vi "run inspection.vi"(7 "Results where TCF match":path[](array[path]), 8 "error in":errorcluster, 9 "Scans[]":T1(array[cluster]), 10 "APG Config":T8, 11 "Programming Data":T2) -> (0 "error out":errorcluster, 2 "Scans[]":T1(array[cluster]), 3 "Inspection passed":bool)   [LabVIEW 2013, in "Manipulate IPF.lvlib"]
uses:
  Manipulate IPF.lvlib
  Settings/type_def/APG Config.ctl
  type_def/files.ctl
  3013/code/Modules/Inspection/Data/Panel_class/type_def/Config File data.ctl
  3013/code/Modules/Inspection/type_def/Pos and Rot.ctl
  3013/code/Modules/Inspection/Data/PCB_class/type_def/PCB Params.ctl
  3013/code/Modules/Inspection/Data/Panel_class/type_def/BarCode Params.ctl
  3013/code/Modules/Barcode Reader/type_def/id.ctl
  <vilib>/addons/WireFlow/_WF_ProgressBar.llb/WindowBehavior.ctl
  <vilib>/addons/WireFlow/_WF_ProgressBar.llb/MessageTextType.ctl
  <vilib>/Utility/sysdir.llb/System Directory Type.ctl
  <vilib>/addons/WireFlow/_WF_ProgressBar.llb/ProgressBar_WireFlow.lvclass
  <userlib>/_OpenG.lib/file/file.llb/Convert File Extension (Path)__ogtk.vi
  <userlib>/_OpenG.lib/file/file.llb/File Exists - Scalar__ogtk.vi
  Mike/APG_mike a3Di.lvlib
  Debug Results/Debug Results.lvlib
  Settings/APG_settings.lvlib
  3013/code/Modules/Inspection/Inspection.lvlib
  3013/code/Modules/Inspection/Data/PCB_class/PCB.lvclass
  3013/code/Modules/Barcode Reader/Barcode Reader.lvlib
  3013/code/Modules/Inspection/Data/Panel_class/Panel.lvclass
  a3Di APG.lvlib
panel:
  out "Array 2":path[](array[path])
  out "Array":path[](array[path])
  out "standard output":string
  out "cmd line":string
  out "Comand debug":string
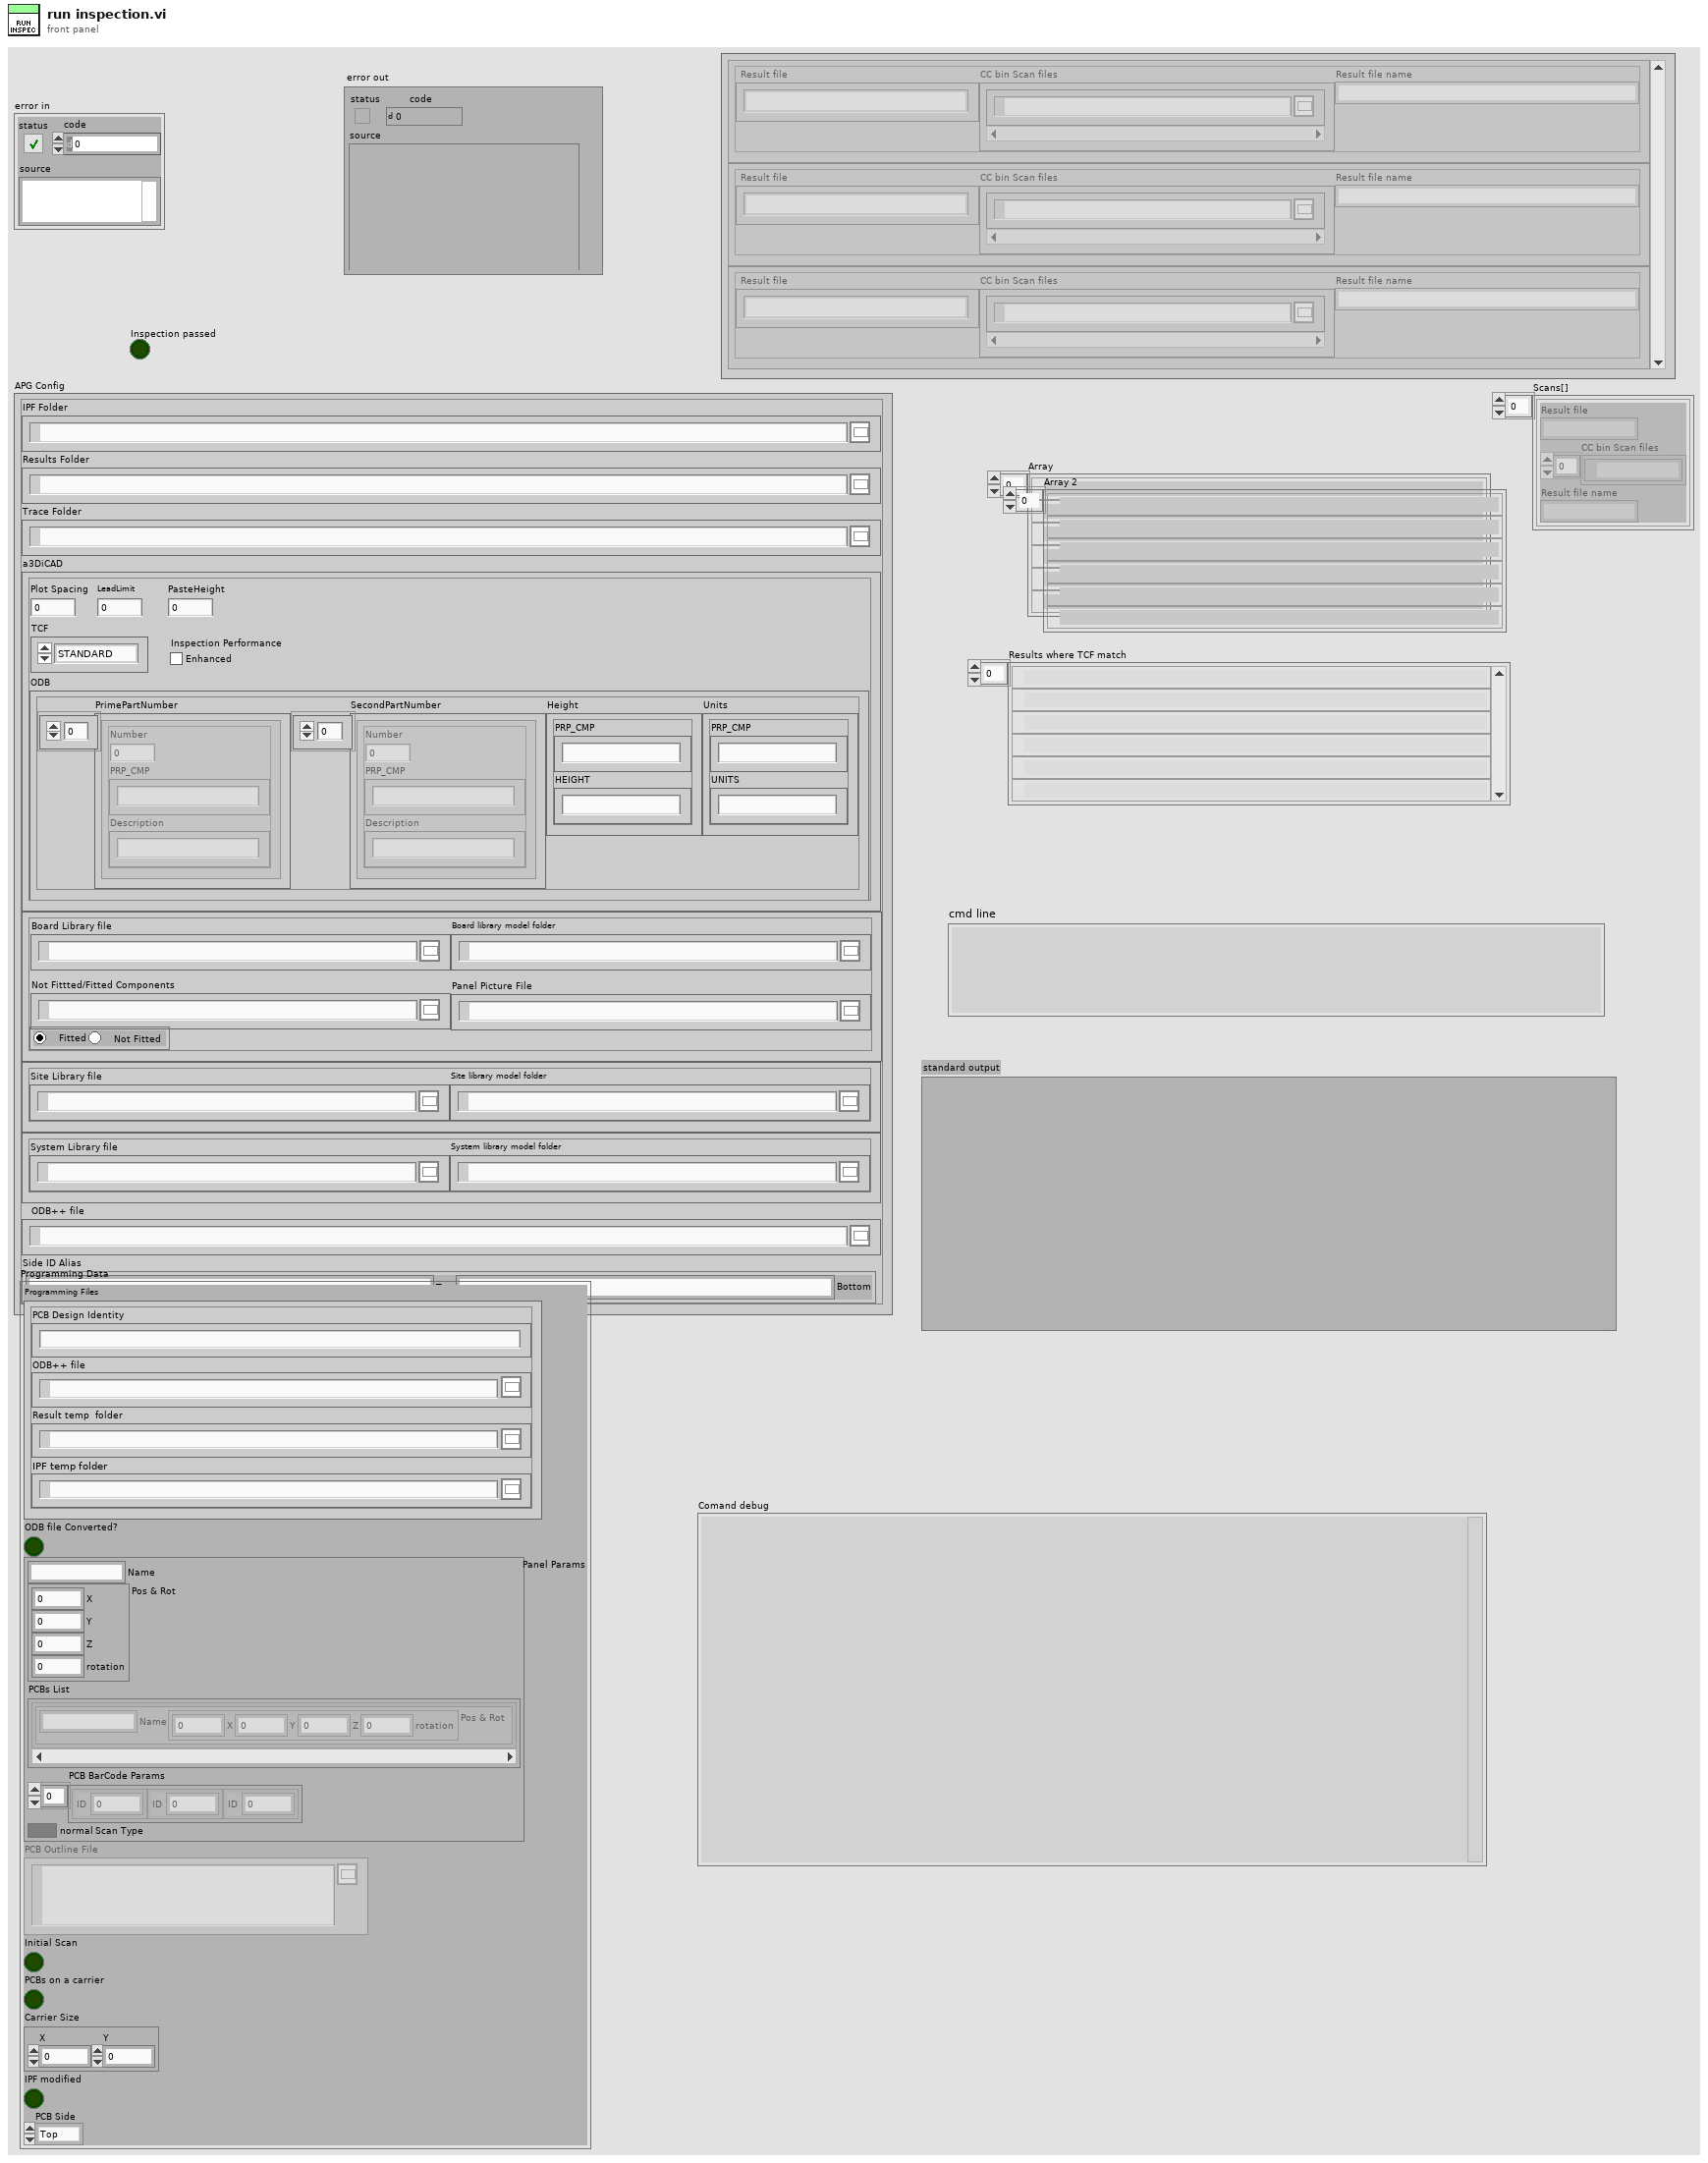
[diagram p1: front panel]
types:
  T1 = cluster{"Result file":string, "CC bin Scan files":path[], "Result file name":string}[]
  T2 = typedef "a3Di APG.lvlib/files.ctl" = cluster{"Programming Files":cluster{"PCB Design Identity":string, "ODB++ file":path, "Result temp  folder":path, "IPF temp folder":path}, "ODB file Converted?":bool, "Panel Params":T3, "PCB Outline File":path, "Initial Scan":bool, "PCBs on a carrier":bool, "Carrier Size":cluster{"X":dbl, "Y":dbl}, "IPF modified":bool, "PCB Side":enum16{"Top", "Bottom"}}
  T3 = typedef "Inspection.lvlib/Panel.lvclass/Config File data.ctl" = cluster{"Name":string, "Pos & Rot":T4, "PCBs List":cluster{"PCB Params":T5}[], "PCB BarCode Params":T6[], "Scan Type":bool}
  T4 = typedef "Inspection.lvlib/Pos and Rot.ctl" = cluster{"X":dbl, "Y":dbl, "Z":dbl, "rotation":dbl}
  T5 = typedef "Inspection.lvlib/PCB.lvclass/PCB Params.ctl" = cluster{"Name":string, "Pos & Rot":T4}
  T6 = typedef "Inspection.lvlib/Panel.lvclass/BarCode Params.ctl" = cluster{"ID":T7}
  T7 = typedef "Barcode Reader.lvlib/id.ctl" = u8
  T8 = typedef "APG_settings.lvlib/APG Config.ctl" = cluster{"IPF Folder":path, "Results Folder":path, "Trace Folder":path, "a3DiCAD":cluster{"Plot Spacing":dbl, "TCF":enum16{"STANDARD", "PASTE", "LEAD"}, "LeadLimit":u32, "a3DiCADDebug":bool, "ODB":cluster{"PrimePartNumber":cluster{"Number":u32, "PRP_CMP":string, "Description":string}[], "SecondPartNumber":cluster{"Number":u32, "PRP_CMP":string, "Description":string}[], "Height":cluster{"PRP_CMP":string, "HEIGHT":string}, "Units":cluster{"PRP_CMP":string, "UNITS":string}}, "PasteHeight":dbl, "Inspection Performance":bool}, "a3DiCADcfg":path, "Board Library":cluster{"Board Library file":path, "Board library model folder":path, "Not Fittted/Fitted Components":path, "Panel Picture File":path, "Components":enum32{"Fitted", "Not Fitted "}}, "Site Library":cluster{"Site Library file":path, "Site library model folder":path}, "System Library":cluster{"System Library file":path, "System library model folder":path}, "ODB++ file":path, "Side ID Alias":cluster{"Top":string, "Bottom":string}}
  T9 = typedef "ProgressBar_WireFlow.lvclass/WindowBehavior.ctl" = enum16{"No change", "Modal", "Floating"}
  T10 = typedef "ProgressBar_WireFlow.lvclass/MessageTextType.ctl" = enum16{"Title", "General", "Current item"}
  T11 = enum16{"open", "replace", "create", "open or create", "replace or create", "replace or create with confirmation"}
  T12 = cluster{"ODB2CPF.exe":path, "TCFToArtworkCPF.exe":path, "TCFToCPFLabels.exe":path, "7z.exe":path, "UpdateTCFLibrary.exe":path, "a3DiPackageTests":path, "Error Codes":path, "TCFToCuboidRefCPF":path, "TCFToArtworkRefCPF":path, "ExtractPKG":path, "ExtractTCFFromODBFileForPKG":path, "OutLineFilterTCFPKG":path, "GenerateLibraryFromTCF":path, "FlipCPF":path, "FlipTCF":path, "TCFToJointBridgeCPF":path, "TCFToJointFR4CPF":path}
  T13 = typedef "System Directory Type.ctl" = i32
  T14 = cluster{"Result file":string, "CC bin Scan files":path[], "Result file name":string}
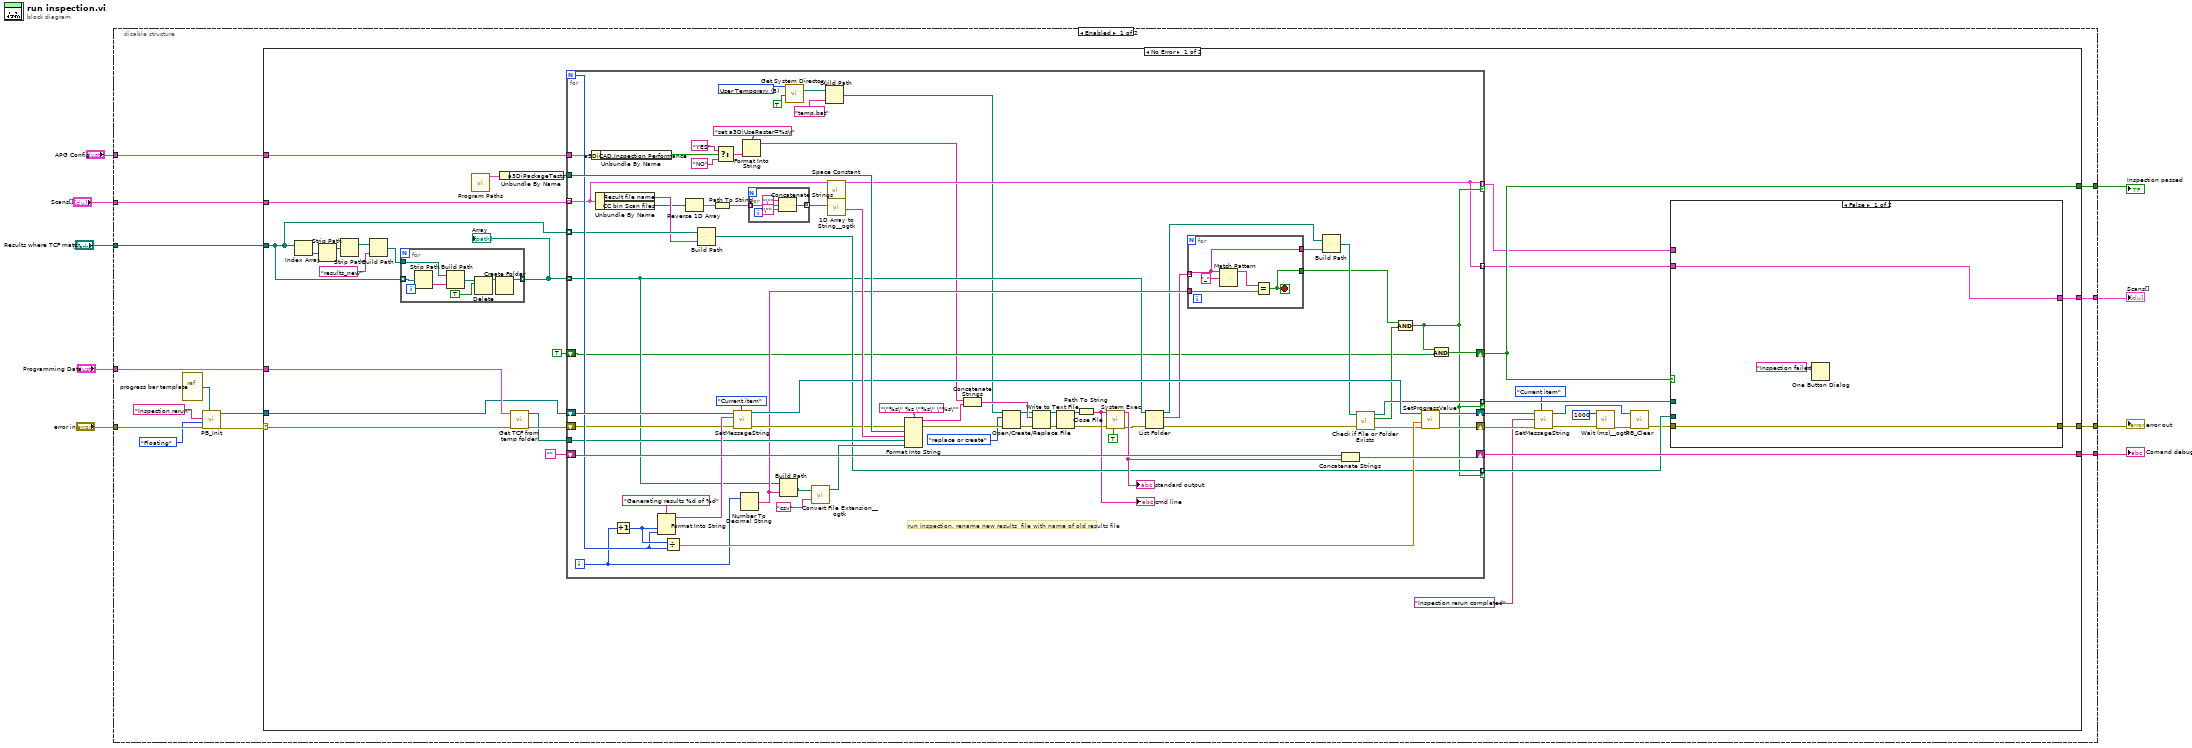
[diagram p0: block diagram]
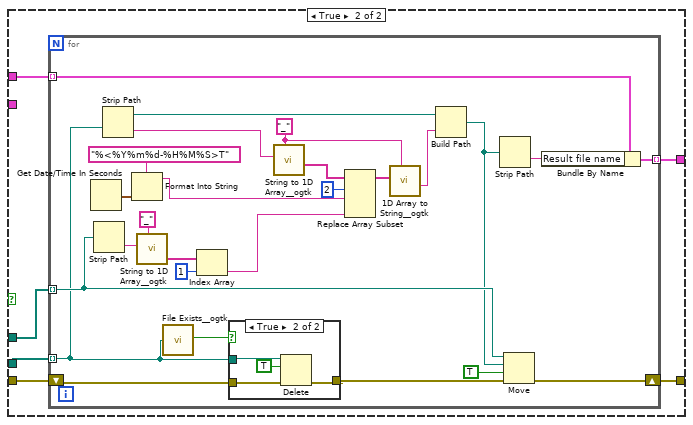
[diagram p2: hidden frame]
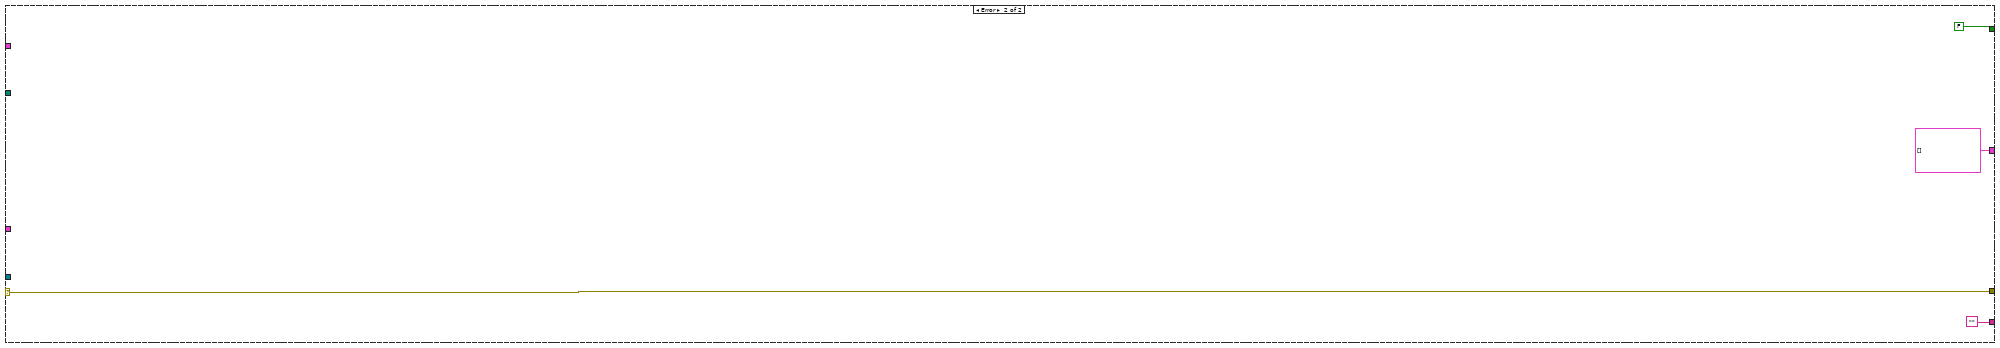
[diagram p4: hidden frame]
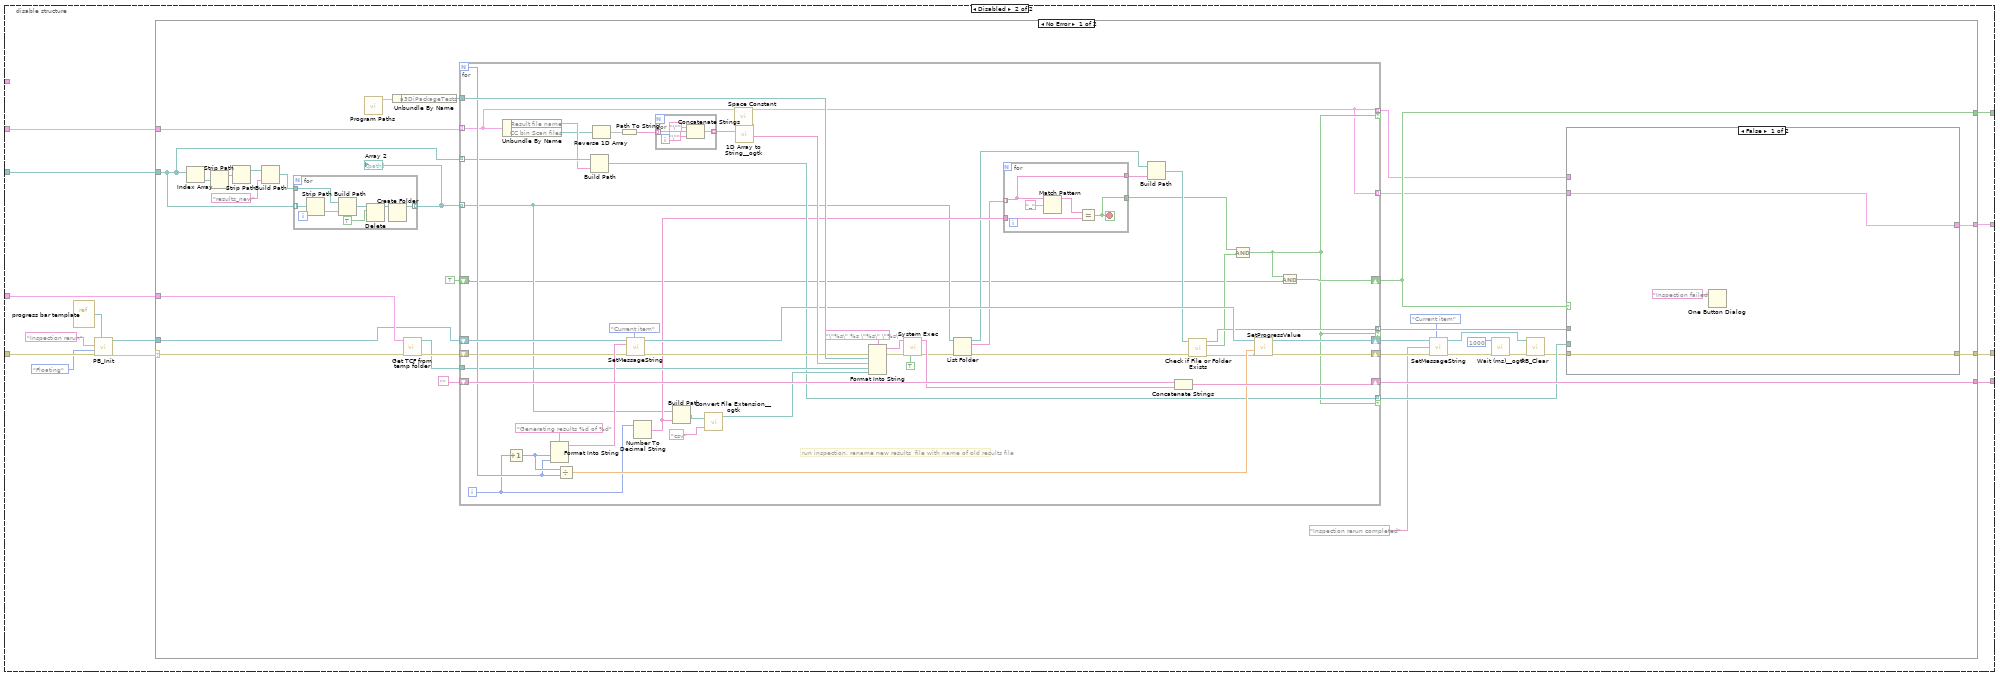
[diagram p5: hidden frame]
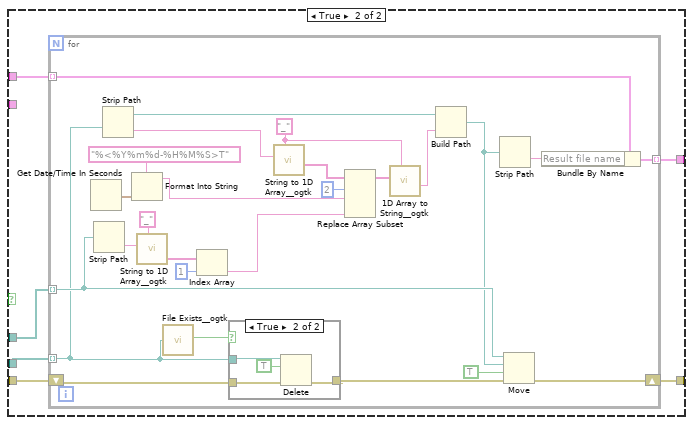
[diagram p6: hidden frame]
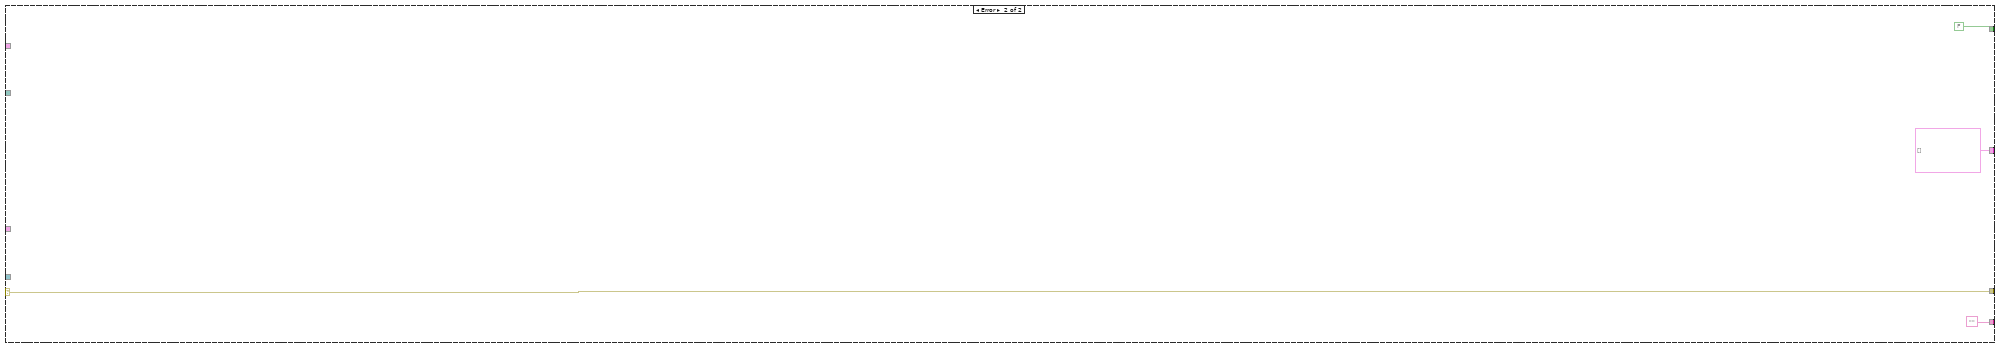
[diagram p8: hidden frame]
diagram:
  n1 = disable-structure shown="Enabled" {
    disable-tunnel: "error in" -> [w16 w195]
    disable-tunnel: [w23 w202] -> w8
    disable-tunnel: "Programming Data" -> [w20 w199]
    disable-tunnel: "APG Config" -> [w10 _]
    disable-tunnel: [w22 w201] -> w5
    disable-tunnel: "Results where TCF match" -> [w21 w200]
    disable-tunnel: "Scans[]" -> [w18 w197]
    disable-tunnel: [w19 w198] -> w2
    disable-tunnel: [w11 w190] -> w1
    frame Enabled {
      n2 = vi-ref "progress bar template.vi"() -> (w14:refnum<vi>)
      n3 = call <vilib>:"PB_Init.vi"("Progress VI"=w14, "error in (no error)"=w16, "Window behavior (No change)"=WindowBehavior."Floating", "title (\"Progress\")"="Inspection rerun" ("title (\"Progress\")")) -> ("error out"=w15:errorcluster, "WF-ProgressBar out"=w17:refnum<class "ProgressBar_WireFlow.lvclass">)  [unwired: 6 in]
      n4 = case shown="No Error" w15 {
        selector: w15 -> [w54 w189]
        tunnel: [w50 w189] -> w23
        tunnel: [w55 ""] -> w22
        tunnel: w21 -> [w33 _]
        tunnel: w18 -> [w28 _]
        tunnel: w20 -> [w51 _]
        tunnel: [w29 FALSE ("exists")] -> w19
        tunnel: w17 -> [w46 _]
        tunnel: [w26 T1 []] -> w11
        tunnel: w10 -> [w24 _]
        frame No Error {
          n5 = Index Array(array=w33) -> (element=w34:path)  [unwired: 1 in]
          n6 = Strip Path(path=w34) -> (stripped path=w37:path)  [unwired: 1 out]
          n7 = Strip Path(path=w37) -> (stripped path=w36:path)  [unwired: 1 out]
          n8 = Build Path(base path=w36, name or relative path="results_new") -> (appended path=w32:path)
          n9 = for {
            tunnel: w33 -> [w65] mode=indexing
            tunnel: w32 -> [w63]
            tunnel: [w62] -> w31 mode=indexing
            n10 = Strip Path(path=w65) -> (name=w64:string)  [unwired: 1 out]
            n11 = Build Path(base path=w63, name or relative path=w64) -> (appended path=w61:path)
            n12 = Delete(path (use dialog)=w61, entire hierarchy (F)=TRUE) -> (deleted path=w60:path)  [unwired: 3 in, 2 out]
            n13 = Create Folder(path (use dialog)=w60) -> (created path=w62:path)  [unwired: 2 in, 2 out]
          }
          "Array" <- w31
          n14 = call "Program Paths.vi"() -> ("Program paths"=w58:T12)  [unwired: 10 in]
          n15 = Unbundle By Name(w58) -> ("a3DiPackageTests"=w57:path)
          n16 = call "Get TCF from temp folder.vi"("error in (no error)"=w54, "Programming Data"=w51) -> ("error out"=w53:errorcluster, "TCF file"=w52:path)  [unwired: 8 in]
          n17 = for {
            N -> [w160]
            tunnel: w57 -> [w175]
            tunnel: w52 -> [w151]
            tunnel: w33 -> [w153] mode=indexing
            shift-right: [w158] -> w44
            shift-left: w53 -> [w154]
            shift-right: [w172] -> w55
            shift-left: "" -> [w174]
            tunnel: w28 -> [w129] mode=indexing
            tunnel: [w145] -> w48 mode=indexing if=w132
            tunnel: [w146] -> w49 mode=indexing if=w132
            shift-right: [w159] -> w43
            shift-left: w46 -> [w164]
            tunnel: w31 -> [w139] mode=indexing
            shift-right: [w147] -> w29
            shift-left: TRUE ("file or folder exists?") -> [w134]
            tunnel: [w129] -> w27 mode=indexing if=w132
            tunnel: [w129] -> w25 mode=indexing
            tunnel: w24 -> [w110]
            i -> [w155]
            w127 = T13 5 items=["User Home"=0, "User Desktop"=1, "User Documents"=2, "User Application Data"=3, "User Preferences"=4, "User Temporary"=5, "Public Documents"=6, "Public Application Data"=7, "Public Preferences"=8, "Public Cache"=13, "System Core Libraries"=9, "System Installed Libraries"=10, "Application Files"=11, "Boot Volume Root"=12] ("system directory type")
            # "run inspection, rename new results  file with name of old results file"
            n18 = Unbundle By Name(w110) -> ("a3DiCAD.Inspection Performance"=w108:bool)
            n19 = Unbundle By Name(w129) -> ("Result file name"=w152:string, "CC bin Scan files"=w131:path[])
            n20 = Increment(x=w155) -> (x+1=w161:i32)
            n21 = Format Into String(format string="Generating results %d of %d", w161, w160) -> (resulting string=w163:string)  [unwired: 2 in, 1 out]
            n22 = Divide(x=w161, y=w160) -> (x/y=w157:dbl)
            n23 = Reverse 1D Array(array=w131) -> (reversed array=w130:path[])
            n24 = Build Path(base path=w153, name or relative path=w152) -> (appended path=w145:path)
            n25 = Path To String(path=w130) -> (string=w171:string[])
            n26 = Select(t="YES", s=w108, f="NO") -> (s? t:f=w107:string)
            n27 = call-dynamic "SetMessageString.vi"("message field"=MessageTextType."Current item", "error in (no error)"=w154, "Message"=w163, "WF-ProgressBar in"=w164) -> ("error out"=w165:errorcluster, "WF-ProgressBar out"=w148:refnum<class "ProgressBar_WireFlow.lvclass">)  [unwired: 6 in]
            n28 = Number To Decimal String(number=w155) -> (decimal integer string=w144:string)  [unwired: 1 in]
            n29 = Format Into String(format string="set a3DiUseRaster=%s\r", w107) -> (resulting string=w112:string)  [unwired: 2 in, 1 out]
            n30 = for {
              tunnel: w171 -> [w184] mode=indexing
              tunnel: [w182] -> w170 mode=indexing
              n31 = Concatenate Strings("\"", w184, "\"") -> (w182:string)
            }
            n32 = Build Path(base path=w139, name or relative path=w144) -> (appended path=w167:path)
            n33 = call <vilib>:"Get System Directory.vi"("create directory if not found? (F)"=TRUE, "system directory type"=w127) -> ("system directory"=w125:path)  [unwired: 9 in]
            n34 = call-poly <userlib>:"Convert File Extension__ogtk.vi"("new ending (none)"="csv", "file name"=w167) -> ("new filename"=w149:path)  [unwired: 1 out]
            n35 = Build Path(base path=w125, name or relative path="temp.bat") -> (appended path=w114:path)
            n36 = call <vilib>:"Space Constant.vi"() -> ("String"=w169:string)
            n37 = call <userlib>:"1D Array to String__ogtk.vi"("delimiter (Tab)"=w169, "Array of Strings"=w170) -> ("delimited string"=w168:string)  [unwired: 9 in]
            n38 = Format Into String(format string="\"%s\" %s \"%s\" \"%s\"", error in=w165, w175, w168, w151, w149) -> (resulting string=w124:string, error out=w116:errorcluster)  [unwired: 1 in]
            n39 = Concatenate Strings(w112, w124) -> (w118:string)
            n40 = Open/Create/Replace File(file path (use dialog)=w114, error in=w116, operation (0:open)=T11."replace or create") -> (refnum out=w115:refnum<file>, error out=w117:errorcluster)  [unwired: 3 in, 1 out]
            n41 = Write to Text File(file (use dialog)=w115, text=w118, error in=w117) -> (refnum out=w119:refnum<file>, error out=w120:errorcluster)  [unwired: 1 in, 1 out]
            n42 = Close File(refnum=w119, error in=w120) -> (path=w121:path, error out=w122:errorcluster)
            n43 = Path To String(path=w121) -> (string=w123:string)
            "cmd line" <- w123
            n44 = call <vilib>:"System Exec.vi"("run minimized? (F)"=TRUE, "error in (no error)"=w122, "command line"=w123) -> ("error out"=w143:errorcluster, "standard output"=w173:string)  [unwired: 5 in, 2 out]
            "standard output" <- w173
            n45 = List Folder(path=w139, error in=w143) -> (path out=w138:path, filenames=w141:string[], error out=w142:errorcluster)  [unwired: 2 in, 1 out]
            n46 = for {
              tunnel: w141 -> [w179] mode=indexing
              tunnel: w144 -> [w178]
              tunnel: [w179] -> w137
              tunnel: [w177] -> w136
              stop <- w177 stop-if-true
              n47 = Match Pattern(string=w179, regular expression="_") -> (before substring=w181:string)  [unwired: 1 in, 3 out]
              n48 = Equal?(x=w181, y=w178) -> (x = y?=w177:bool)
            }
            n49 = Build Path(base path=w138, name or relative path=w137) -> (appended path=w140:path)
            n50 = Concatenate Strings(w174, w173) -> (w172:string)
            n51 = call <vilib>:"Check if File or Folder Exists.vi"("error in (no error)"=w142, "path"=w140) -> ("error out"=w150:errorcluster, "file or folder exists?"=w135:bool, "dup path"=w146:path)  [unwired: 7 in]
            n52 = Compound Arithmetic op=AND(w136, w135) -> (w132:bool)
            n53 = call-dynamic "SetProgressValue.vi"("error in (no error)"=w150, "Value"=w157, "WF-ProgressBar in"=w148) -> ("error out"=w158:errorcluster, "WF-ProgressBar out"=w159:refnum<class "ProgressBar_WireFlow.lvclass">)  [unwired: 6 in, 1 out]
            n54 = And(x=w132, y=w134) -> (x .and. y?=w147:bool)
          }
          n55 = call-dynamic "SetMessageString.vi"("message field"=MessageTextType."Current item", "error in (no error)"=w44, "Message"="Inspection rerun completed", "WF-ProgressBar in"=w43) -> ("error out"=w39:errorcluster, "WF-ProgressBar out"=w38:refnum<class "ProgressBar_WireFlow.lvclass">)  [unwired: 6 in]
          n56 = call <userlib>:"Wait (ms)__ogtk.vi"("error in (no error)"=w39, "milliseconds to wait"=u32 1000) -> ("error out"=w40:errorcluster)  [unwired: 8 in, 1 out]
          n57 = call-dynamic "PB_Clear.vi"("error in (no error)"=w40, "WF-ProgressBar in"=w38) -> ("error out"=w47:errorcluster)  [unwired: 8 in, 1 out]
          n58 = case shown="False" w29 {
            tunnel: w47 -> [w67 w74]
            tunnel: [w67 w71] -> w50
            tunnel: w49 -> [_ w73]
            tunnel: w48 -> [_ w72]
            tunnel: w27 -> [_ w70]
            tunnel: [w66 w69] -> w26
            tunnel: w25 -> [w66 _]
            frame False {
              n59 = One Button Dialog(message="Inspection failed") -> ()  [unwired: 1 in, 1 out]
            }
            frame True {
              n60 = for {
                tunnel: w73 -> [w87] mode=indexing
                tunnel: w72 -> [w84] mode=indexing
                shift-right: [w100] -> w71
                shift-left: w74 -> [w85]
                tunnel: w70 -> [w78] mode=indexing
                tunnel: [w77] -> w69 mode=indexing
                w88 = "_"
                n61 = Get Date/Time In Seconds() -> (seconds since 1Jan1904=w81:timestamp)
                n62 = Strip Path(path=w87) -> (name=w92:string)  [unwired: 1 out]
                n63 = Strip Path(path=w84) -> (stripped path=w93:path, name=w95:string)
                n64 = Format Into String(format string="%<%Y%m%d-%H%M%S>T", w81) -> (resulting string=w80:string)  [unwired: 2 in, 1 out]
                n65 = call <userlib>:"String to 1D Array__ogtk.vi"("delimiter (Tab)"="_", "string"=w92) -> ("Array of Strings"=w91:string[])  [unwired: 9 in]
                n66 = call-poly <userlib>:"File Exists__ogtk.vi"("file path"=w84) -> ("exists"=w83:bool)  [unwired: 6 in, 1 out]
                n67 = Index Array(array=w91, index=1) -> (element=w82:string)
                n68 = case shown="True" w83 {
                  tunnel: [w101 w104] -> w86
                  tunnel: w85 -> [w101 w105]
                  tunnel: w84 -> [_ w103]
                  frame False {
                  }
                  frame True {
                    n69 = Delete(path (use dialog)=w103, entire hierarchy (F)=TRUE, error in=w105) -> (error out=w104:errorcluster)  [unwired: 2 in, 2 out]
                  }
                }
                n70 = call <userlib>:"String to 1D Array__ogtk.vi"("delimiter (Tab)"=w88, "string"=w95) -> ("Array of Strings"=w98:string[])  [unwired: 9 in]
                n71 = Replace Array Subset(array=w98, new element #1=w80, index #1=2 ("index"), new element #2=w82) -> (w96:string[])  [unwired: 1 in]
                n72 = call <userlib>:"1D Array to String__ogtk.vi"("delimiter (Tab)"=w88, "Array of Strings"=w96) -> ("delimited string"=w94:string)  [unwired: 9 in]
                n73 = Build Path(base path=w93, name or relative path=w94) -> (appended path=w75:path)
                n74 = Strip Path(path=w75) -> (name=w76:string)  [unwired: 1 out]
                n75 = Move(source path=w87, error in=w86, 9:TRUE ("overwrite (F)"), 10:w75) -> (error out=w100:errorcluster)  [unwired: 1 in, 2 out]
                n76 = Bundle By Name(cluster=w78, "Result file name"=w76) -> (w77:T14)
              }
            }
          }
        }
        frame Error {
        }
      }
    }
    frame Disabled {
      n77 = vi-ref "progress bar template.vi"() -> (w193:refnum<vi>)
      n78 = call <vilib>:"PB_Init.vi"("Progress VI"=w193, "error in (no error)"=w195, "Window behavior (No change)"=WindowBehavior."Floating", "title (\"Progress\")"="Inspection rerun" ("title (\"Progress\")")) -> ("error out"=w194:errorcluster, "WF-ProgressBar out"=w196:refnum<class "ProgressBar_WireFlow.lvclass">)  [unwired: 6 in]
      n79 = case shown="No Error" w194 {
        selector: w194 -> [w232 w346]
        tunnel: [w228 w346] -> w202
        tunnel: [w233 ""] -> w201
        tunnel: w200 -> [w211 _]
        tunnel: w197 -> [w206 _]
        tunnel: w199 -> [w229 _]
        tunnel: [w207 FALSE ("exists")] -> w198
        tunnel: w196 -> [w224 _]
        tunnel: [w204 T1 []] -> w190
        frame No Error {
          n80 = Index Array(array=w211) -> (element=w212:path)  [unwired: 1 in]
          n81 = Strip Path(path=w212) -> (stripped path=w215:path)  [unwired: 1 out]
          n82 = Strip Path(path=w215) -> (stripped path=w214:path)  [unwired: 1 out]
          n83 = Build Path(base path=w214, name or relative path="results_new") -> (appended path=w210:path)
          n84 = for {
            tunnel: w211 -> [w243] mode=indexing
            tunnel: w210 -> [w241]
            tunnel: [w240] -> w209 mode=indexing
            n85 = Strip Path(path=w243) -> (name=w242:string)  [unwired: 1 out]
            n86 = Build Path(base path=w241, name or relative path=w242) -> (appended path=w239:path)
            n87 = Delete(path (use dialog)=w239, entire hierarchy (F)=TRUE) -> (deleted path=w238:path)  [unwired: 3 in, 2 out]
            n88 = Create Folder(path (use dialog)=w238) -> (created path=w240:path)  [unwired: 2 in, 2 out]
          }
          "Array 2" <- w209
          n89 = call "Program Paths.vi"() -> ("Program paths"=w236:T12)  [unwired: 10 in]
          n90 = Unbundle By Name(w236) -> ("a3DiPackageTests"=w235:path)
          n91 = call "Get TCF from temp folder.vi"("error in (no error)"=w232, "Programming Data"=w229) -> ("error out"=w231:errorcluster, "TCF file"=w230:path)  [unwired: 8 in]
          n92 = for {
            N -> [w315]
            tunnel: w235 -> [w330]
            tunnel: w230 -> [w306]
            tunnel: w211 -> [w308] mode=indexing
            shift-right: [w313] -> w222
            shift-left: w231 -> [w309]
            shift-right: [w327] -> w233
            shift-left: "" -> [w329]
            tunnel: w206 -> [w284] mode=indexing
            tunnel: [w300] -> w226 mode=indexing if=w287
            tunnel: [w301] -> w227 mode=indexing if=w287
            shift-right: [w314] -> w221
            shift-left: w224 -> [w319]
            tunnel: w209 -> [w294] mode=indexing
            shift-right: [w302] -> w207
            shift-left: TRUE ("file or folder exists?") -> [w289]
            tunnel: [w284] -> w205 mode=indexing if=w287
            tunnel: [w284] -> w203 mode=indexing
            i -> [w310]
            # "run inspection, rename new results  file with name of old results file"
            n93 = Unbundle By Name(w284) -> ("Result file name"=w307:string, "CC bin Scan files"=w286:path[])
            n94 = Increment(x=w310) -> (x+1=w316:i32)
            n95 = Format Into String(format string="Generating results %d of %d", w316, w315) -> (resulting string=w318:string)  [unwired: 2 in, 1 out]
            n96 = Divide(x=w316, y=w315) -> (x/y=w312:dbl)
            n97 = Build Path(base path=w308, name or relative path=w307) -> (appended path=w300:path)
            n98 = Reverse 1D Array(array=w286) -> (reversed array=w285:path[])
            n99 = Path To String(path=w285) -> (string=w326:string[])
            n100 = call-dynamic "SetMessageString.vi"("message field"=MessageTextType."Current item", "error in (no error)"=w309, "Message"=w318, "WF-ProgressBar in"=w319) -> ("error out"=w320:errorcluster, "WF-ProgressBar out"=w303:refnum<class "ProgressBar_WireFlow.lvclass">)  [unwired: 6 in]
            n101 = Number To Decimal String(number=w310) -> (decimal integer string=w299:string)  [unwired: 1 in]
            n102 = for {
              tunnel: w326 -> [w341] mode=indexing
              tunnel: [w339] -> w325 mode=indexing
              n103 = Concatenate Strings("\"", w341, "\"") -> (w339:string)
            }
            n104 = Build Path(base path=w294, name or relative path=w299) -> (appended path=w322:path)
            n105 = call-poly <userlib>:"Convert File Extension__ogtk.vi"("new ending (none)"="csv", "file name"=w322) -> ("new filename"=w304:path)  [unwired: 1 out]
            n106 = call <vilib>:"Space Constant.vi"() -> ("String"=w324:string)
            n107 = call <userlib>:"1D Array to String__ogtk.vi"("delimiter (Tab)"=w324, "Array of Strings"=w325) -> ("delimited string"=w323:string)  [unwired: 9 in]
            n108 = Format Into String(format string="\"%s\" %s \"%s\" \"%s\"", error in=w320, w330, w323, w306, w304) -> (resulting string=w332:string, error out=w333:errorcluster)  [unwired: 1 in]
            n109 = call <vilib>:"System Exec.vi"("run minimized? (F)"=TRUE, "error in (no error)"=w333, "command line"=w332) -> ("error out"=w298:errorcluster, "standard output"=w328:string)  [unwired: 5 in, 2 out]
            n110 = List Folder(path=w294, error in=w298) -> (path out=w293:path, filenames=w296:string[], error out=w297:errorcluster)  [unwired: 2 in, 1 out]
            n111 = for {
              tunnel: w296 -> [w336] mode=indexing
              tunnel: w299 -> [w335]
              tunnel: [w336] -> w292
              tunnel: [w334] -> w291
              stop <- w334 stop-if-true
              n112 = Match Pattern(string=w336, regular expression="_") -> (before substring=w338:string)  [unwired: 1 in, 3 out]
              n113 = Equal?(x=w338, y=w335) -> (x = y?=w334:bool)
            }
            n114 = Build Path(base path=w293, name or relative path=w292) -> (appended path=w295:path)
            n115 = Concatenate Strings(w329, w328) -> (w327:string)
            n116 = call <vilib>:"Check if File or Folder Exists.vi"("error in (no error)"=w297, "path"=w295) -> ("error out"=w305:errorcluster, "file or folder exists?"=w290:bool, "dup path"=w301:path)  [unwired: 7 in]
            n117 = Compound Arithmetic op=AND(w291, w290) -> (w287:bool)
            n118 = call-dynamic "SetProgressValue.vi"("error in (no error)"=w305, "Value"=w312, "WF-ProgressBar in"=w303) -> ("error out"=w313:errorcluster, "WF-ProgressBar out"=w314:refnum<class "ProgressBar_WireFlow.lvclass">)  [unwired: 6 in, 1 out]
            n119 = And(x=w287, y=w289) -> (x .and. y?=w302:bool)
          }
          n120 = call-dynamic "SetMessageString.vi"("message field"=MessageTextType."Current item", "error in (no error)"=w222, "Message"="Inspection rerun completed", "WF-ProgressBar in"=w221) -> ("error out"=w217:errorcluster, "WF-ProgressBar out"=w216:refnum<class "ProgressBar_WireFlow.lvclass">)  [unwired: 6 in]
          n121 = call <userlib>:"Wait (ms)__ogtk.vi"("error in (no error)"=w217, "milliseconds to wait"=u32 1000) -> ("error out"=w218:errorcluster)  [unwired: 8 in, 1 out]
          n122 = call-dynamic "PB_Clear.vi"("error in (no error)"=w218, "WF-ProgressBar in"=w216) -> ("error out"=w225:errorcluster)  [unwired: 8 in, 1 out]
          n123 = case shown="False" w207 {
            tunnel: w225 -> [w245 w252]
            tunnel: [w245 w249] -> w228
            tunnel: w227 -> [_ w251]
            tunnel: w226 -> [_ w250]
            tunnel: w205 -> [_ w248]
            tunnel: [w244 w247] -> w204
            tunnel: w203 -> [w244 _]
            frame False {
              n124 = One Button Dialog(message="Inspection failed") -> ()  [unwired: 1 in, 1 out]
            }
            frame True {
              n125 = for {
                tunnel: w251 -> [w265] mode=indexing
                tunnel: w250 -> [w262] mode=indexing
                shift-right: [w278] -> w249
                shift-left: w252 -> [w263]
                tunnel: w248 -> [w256] mode=indexing
                tunnel: [w255] -> w247 mode=indexing
                w266 = "_"
                n126 = Get Date/Time In Seconds() -> (seconds since 1Jan1904=w259:timestamp)
                n127 = Strip Path(path=w265) -> (name=w270:string)  [unwired: 1 out]
                n128 = Strip Path(path=w262) -> (stripped path=w271:path, name=w273:string)
                n129 = Format Into String(format string="%<%Y%m%d-%H%M%S>T", w259) -> (resulting string=w258:string)  [unwired: 2 in, 1 out]
                n130 = call <userlib>:"String to 1D Array__ogtk.vi"("delimiter (Tab)"="_", "string"=w270) -> ("Array of Strings"=w269:string[])  [unwired: 9 in]
                n131 = call-poly <userlib>:"File Exists__ogtk.vi"("file path"=w262) -> ("exists"=w261:bool)  [unwired: 6 in, 1 out]
                n132 = Index Array(array=w269, index=1) -> (element=w260:string)
                n133 = case shown="True" w261 {
                  tunnel: [w279 w282] -> w264
                  tunnel: w263 -> [w279 w283]
                  tunnel: w262 -> [_ w281]
                  frame False {
                  }
                  frame True {
                    n134 = Delete(path (use dialog)=w281, entire hierarchy (F)=TRUE, error in=w283) -> (error out=w282:errorcluster)  [unwired: 2 in, 2 out]
                  }
                }
                n135 = call <userlib>:"String to 1D Array__ogtk.vi"("delimiter (Tab)"=w266, "string"=w273) -> ("Array of Strings"=w276:string[])  [unwired: 9 in]
                n136 = Replace Array Subset(array=w276, new element #1=w258, index #1=2 ("index"), new element #2=w260) -> (w274:string[])  [unwired: 1 in]
                n137 = call <userlib>:"1D Array to String__ogtk.vi"("delimiter (Tab)"=w266, "Array of Strings"=w274) -> ("delimited string"=w272:string)  [unwired: 9 in]
                n138 = Build Path(base path=w271, name or relative path=w272) -> (appended path=w253:path)
                n139 = Strip Path(path=w253) -> (name=w254:string)  [unwired: 1 out]
                n140 = Move(source path=w265, error in=w264, 9:TRUE ("overwrite (F)"), 10:w253) -> (error out=w278:errorcluster)  [unwired: 1 in, 2 out]
                n141 = Bundle By Name(cluster=w256, "Result file name"=w254) -> (w255:T14)
              }
            }
          }
        }
        frame Error {
        }
      }
    }
  }
  "error out" <- w8
  "Comand debug" <- w5
  "Inspection passed" <- w2
  "Scans[]" <- w1
